vi "Agilent 428X Series Continual Measurement.vi"(6 "stop":bool, 7 "Voltage Level (V)(1.0V)":dbl=1.0 min=0.0 max=20.0 step=0.1 format="%.4f", 8 "error in (no error)":errorcluster, 9 "Freq Value (Hz)(1.0 MHz)":dbl=1000020.0 min=20.0 max=30000000.0 step=100000.0 format="%.2e", 10 "Imp Type (0: CPD)":u32(ring) items=["CPD", "CPQ", "CPG", "CPRP", "CSD", "CSQ", "CSRS", "LPQ", "LPD", "LPG", "LPRP", "LSD", "LSQ", "LSRS", "RX", "ZTD", "ZTR", "GB", "YTD", "YTR"], 11 "VISA resource name":refnum<visa-resource-name>) -> (0 "error out":errorcluster, 1 "Secondary Value":dbl format="%^.4e", 2 "Primary Value":dbl format="%^.4e", 3 "VISA resource name out":refnum<visa-resource-name>, 4 "Data Status":bool=TRUE)   [LabVIEW 2015]
doc: "This VI is an example of how to use the HP428XA subVIs programmatically. This VI first configures a measurement, sets triggering, then takes continual measurements until is stopped.\n\nThis VI is fully compatible with Application Function VI.\n\nThis function demonstrate one type of impedance measurement that can be made with the HP428XA and it accessories. In this example a 220 pF ceramic capacitor will be measured under the following conditions.\n\n DUT:\n 220 pF ceramic capacitor\n (HP Part Number 0160-4812)\n\n Measurement Conditions: \n \n Function: Cp-D\n Frequency: 1.0 MHz\n Test Signal Level: 1.0 V\n \n Equipment Required:\n\n HP 16047C Test Fixture\n Shorting bar (HP Part Number 5000-4226) or equivalent\n\nNote:\nFor more details see to the operation manual in Chapter 3."
uses:
  <instrlib>/Agilent 428X Series/Agilent 428X Series.lvlib
panel:
  # "© Copyright 2005 National Instruments Corporation.  All Rights Reserved."
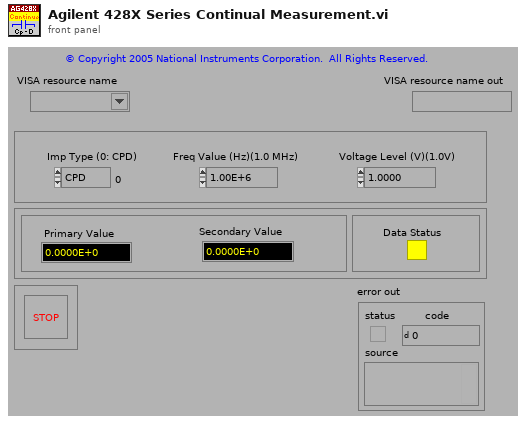
[diagram p1: front panel]
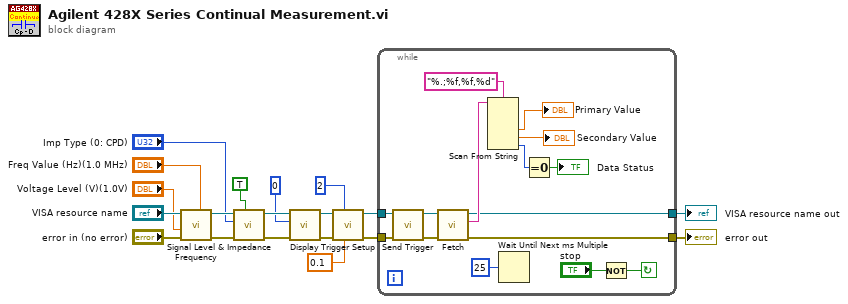
[diagram p0: block diagram]
diagram:
  n1 = call <instrlib>:"Signal Level & Frequency.vi"("Frequency Value (Hz) (100KHz)"="Freq Value (Hz)(1.0 MHz)", "error in (no error)"="error in (no error)", "Voltage Level (V) (5mV)"="Voltage Level (V)(1.0V)", "VISA resource name"="VISA resource name") -> ("error out"=w10:errorcluster, "VISA resource name out"=w19:refnum<visa-resource-name>)  [unwired: 6 in]
  n2 = call <instrlib>:"Impedance.vi"("Auto Range (F: Off)"=TRUE ("Auto Range (Off:F)"), "error in (no error)"=w10, "Imp Type (0: CPD)"="Imp Type (0: CPD)", "VISA resource name"=w19) -> ("error out"=w11:errorcluster, "VISA resource name out"=w18:refnum<visa-resource-name>)  [unwired: 6 in]
  n3 = call <instrlib>:"Display.vi"("error in (no error)"=w11, "Display Page (0: Measurement)"=u32 0 ("Display Page (Measurment:0)"), "VISA resource name"=w18) -> ("error out"=w12:errorcluster, "VISA resource name out"=w17:refnum<visa-resource-name>)  [unwired: 7 in]
  n4 = call <instrlib>:"Trigger Setup.vi"("Delay Value (s) (0.0)"=0.1, "Trigger Source (0: Internal)"=u32 2 ("Trigger Source (Internal:0)"), "error in (no error)"=w12, "VISA resource name"=w17) -> ("error out"=w13:errorcluster, "VISA resource name out"=w16:refnum<visa-resource-name>)  [unwired: 6 in]
  n5 = while {
    tunnel: w16 -> [w25]
    tunnel: [w27] -> w15
    tunnel: [w28] -> w14
    tunnel: w13 -> [w29]
    stop <- w23 continue-if-true
    n6 = call <instrlib>:"Send Trigger.vi"("error in (no error)"=w29, "VISA resource name"=w25) -> ("error out"=w34:errorcluster, "VISA resource name out"=w26:refnum<visa-resource-name>)  [unwired: 8 in]
    n7 = call <instrlib>:"Fetch.vi"("error in (no error)"=w34, "VISA resource name"=w26) -> ("error out"=w28:errorcluster, "Returned Data"=w30:string, "VISA resource name out"=w27:refnum<visa-resource-name>)  [unwired: 7 in]
    n8 = Scan From String(format string="%.;%f,%f,%d", input string=w30) -> (output 1=→"Primary Value":dbl, output 2=→"Secondary Value":dbl, output 3=w33:i32)  [unwired: 5 in, 3 out]
    n9 = Wait Until Next ms Multiple(millisecond multiple=u32 25) -> ()  [unwired: 1 out]
    n10 = Equal To 0?(x=w33) -> (x = 0?=→"Data Status":bool)
    n11 = Not(x="stop") -> (.not. x?=w23:bool)
  }
  "VISA resource name out" <- w15
  "error out" <- w14
